vi "Initialise.vi"(8 "error in (no error)":errorcluster, 11 "DAQ Types in":refnum<class "DAQ Types.lvclass">) -> (0 "error out":errorcluster, 2 "Status":string, 3 "DAQ Types out":refnum<class "DAQ Types.lvclass">)   [LabVIEW 2020, in "DAQ Types.lvclass"]
uses:
  DAQ Types.lvclass
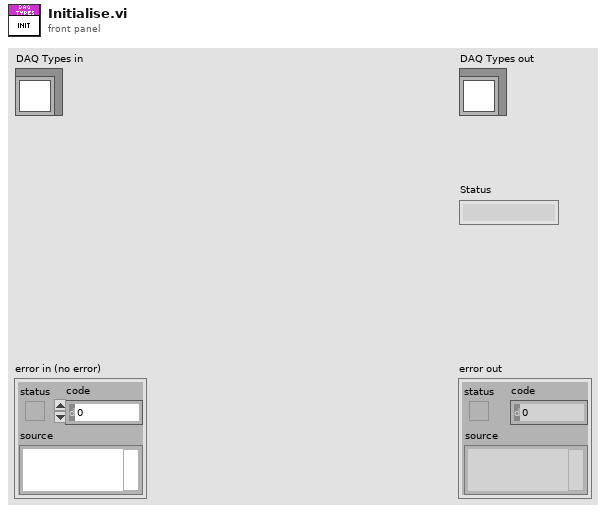
[diagram p1: front panel]
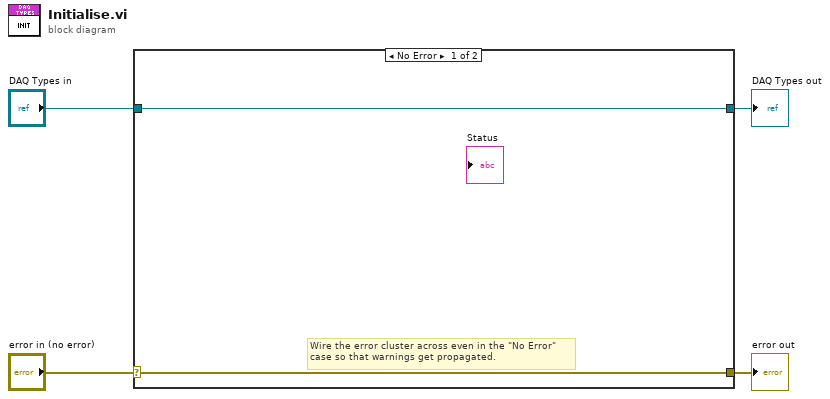
[diagram p0: block diagram]
diagram:
  n1 = case shown="No Error" "error in (no error)" {
    selector: "error in (no error)" -> [w5 w8]
    tunnel: [w5 w8] -> w3
    tunnel: [w6 w7] -> w1
    tunnel: "DAQ Types in" -> [w6 w7]
    frame No Error {
      # "Wire the error cluster across even in the \"No Error\"\ncase so that warnings get propagated."
    }
    frame Error {
    }
  }
  "error out" <- w3
  "DAQ Types out" <- w1
